vi "PXF4_get_manual_MV.vi"(8 "error in":errorcluster, 11 "Modbus Master in":refnum<class "Modbus Master.lvclass">) -> (0 "error out":errorcluster, 1 "onoff":bool, 2 "MV":u8, 3 "Modbus Master out":refnum<class "Modbus Master.lvclass">)   [LabVIEW 2019]
uses:
  <vilib>/NI/Modbus Library/API/Master/Modbus Master.lvclass
panel:
  out "register values":u16[](array[numeric])
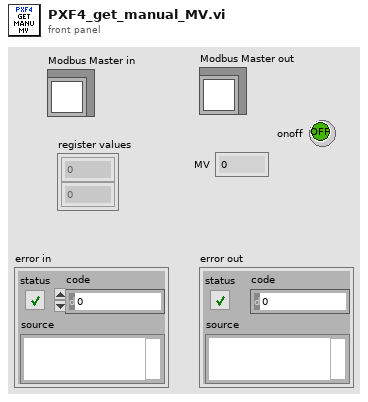
[diagram p1: front panel]
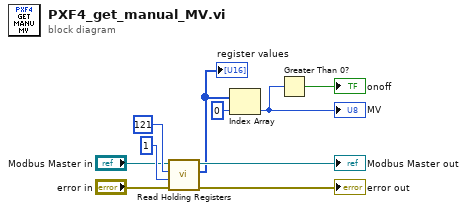
[diagram p0: block diagram]
diagram:
  n1 = call-dynamic "Read Holding Registers.vi"("error in"="error in", "number of inputs"=u16 1, "starting address"=u16 121, "Modbus master in"="Modbus Master in") -> ("error out"=→"error out":errorcluster, "register values"=w7:u16[], "Modbus master out"=→"Modbus Master out":refnum<class "Modbus Master.lvclass">)  [unwired: 5 in]
  "register values" <- w7
  n2 = Index Array(array=w7, index=0) -> (element=w2:u16)
  "MV" <- w2
  n3 = Greater Than 0?(x=w2) -> (x > 0?=→"onoff":bool)
